vi "GetOscilloscopesNames[].vi"(8 "error in (no error)":errorcluster) -> (0 "error IO":errorcluster, 3 "OscilloscopesNames[]":string[](array[string]))   [LabVIEW 2013]
doc: "Load from the database the list of all the devices registered as \"Oscilloscope\""
uses:
  Shared/MySQL/Preset Query Enum.ctl
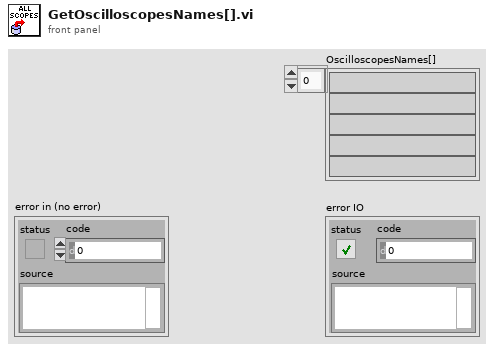
[diagram p1: front panel]
types:
  T1 = typedef "Preset Query Enum.ctl" = enum16{"Get Locations", "Get all IPs and MACs", "Get classes", "Get expt variables to set at scanstart for particular device", "Get expt devices and variables with start values", "Get expt devices and variables (with data to get)", "Get expt devices with data to get", "Get Expt devices and GUIs", "Get all devices basic properties", "Get Virtual Devices Core Info", "Get Expt names", "Get experiment basic properties", "Get experiment alarm variables", "Get MC Ports", "Get device network comm port", "Get devicetype lvclass path", "Get basic device properties", "Get Init Order", "Get all setable variables of a device", "Get device variable aliases", "Get force values of all settable variables", "Get all variables of a devicetype", "Get all variables of a device", "Get plotter details", "Get Saved Scans", "Get Scan Info", "GetGeneralGUIs", "Get expt for plotter", "Get plotter IDs from expt", "Get all devices", "Get all Virtual Devices", "Get all aliases", "Get variable and device info for Virtual Device", "GetItemLocatorIP", "Get IPs for GUIs", "Get DeviceType from Device", "GetLocalPortRange", "GetDevicePresetVariables", "Get Device Configuration", "GetAllPresetNames", "GetAllConfigurationNames", "GetPresetDeviceNames"}
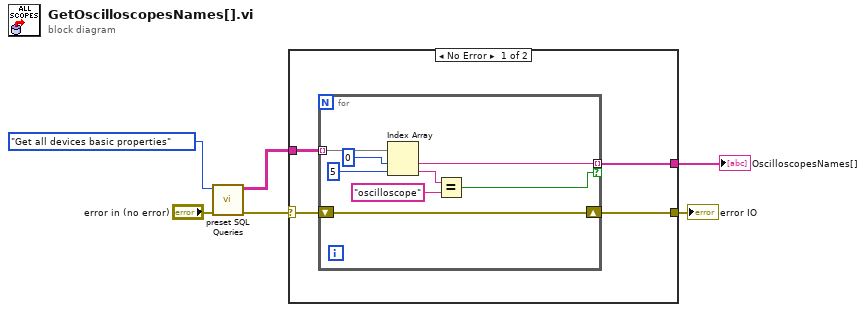
[diagram p0: block diagram]
diagram:
  n1 = call "preset SQL Queries.vi"("error in (no error)"="error in (no error)", "Preset Query"=Preset_Query_Enum."Get all devices basic properties") -> ("error out"=w2:errorcluster, "data"=w5:string[][])  [unwired: 7 in, 1 out]
  n2 = case shown="No Error" w2 {
    selector: w2 -> [w7 w19]
    tunnel: w5 -> [w10 _]
    tunnel: [w9 _] -> w3
    tunnel: [w8 w19] -> w1
    frame No Error {
      n3 = for {
        tunnel: w10 -> [w18] mode=indexing
        tunnel: [w13] -> w9 mode=indexing if=w12
        shift-right: [w11] -> w8
        shift-left: w7 -> [w11]
        n4 = Index Array(array=w18, index #1=0 ("index"), index #2=5 ("index")) -> (element #1=w13:string, element #2=w16:string)
        n5 = Equal?(x=w16, y="oscilloscope") -> (x = y?=w12:bool)
      }
    }
    frame Error {
    }
  }
  "OscilloscopesNames[]" <- w3
  "error IO" <- w1
